vi "Initialize.vi"(8 "error in (no error)":errorcluster, 10 "Name":string, 11 "Filter Wheel Simulator in":refnum<class "Filter Wheel Simulator.lvclass">) -> (0 "error out":errorcluster, 3 "Filter Wheel Simulator out":refnum<class "Filter Wheel Simulator.lvclass">)   [LabVIEW 2021, in "Filter Wheel Simulator.lvclass"]
uses:
  Filter Wheel Simulator.lvclass
  Filter Wheel cluster Simulated Status.ctl
  Filter Wheel Simulator.lvclass/Filter Wheel Simulator.ctl
  Filter Wheel Object/Filter Wheel.lvclass
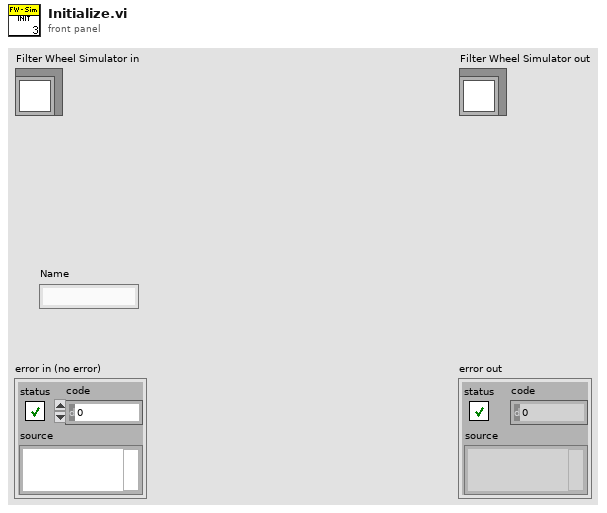
[diagram p1: front panel]
types:
  T1 = typedef "Filter Wheel Simulator.lvclass/Filter Wheel cluster Simulated Status.ctl" = cluster{"Move Start Time":timestamp, "Moving?":bool, "Target Pos":dbl, "Direction":bool}
  T2 = typedef "Filter Wheel.lvclass/Filter Wheel configuration.ctl" = cluster{"Num Wheels":i32, "Filters":T3[], "Invalid Combinations":i32[][], "Addr":refnum<visa-resource-name>, "Name":string, "Simulate":bool, "Homing Parameters":T4, "Default Speed":u16}
  T3 = typedef "Filter Wheel.lvclass/Filter Wheel Details.ctl" = cluster{"Names":string[], "Relative Position":i32[], "Wheel Name":string}
  T4 = typedef "Filter Wheel Arduino Homing cluster.ctl" = cluster{"Direction (F: CW)":bool, "Speed":i32, "Accel":i32, "Min Distance":i32, "Short Leg":i32, "Error Cnts":i32}
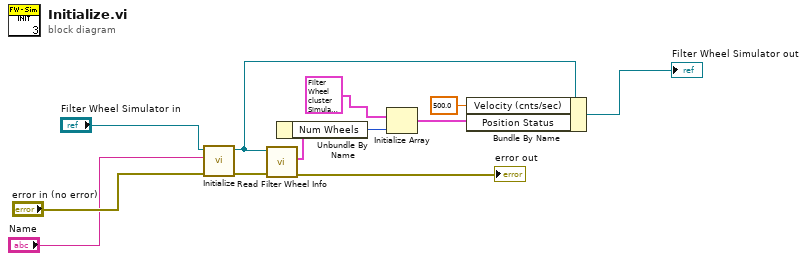
[diagram p0: block diagram]
diagram:
  n1 = call-parent "Initialize.vi"("error in (no error)"="error in (no error)", "Name"="Name", "Filter Wheel in"="Filter Wheel Simulator in") -> ("error out"=w7:errorcluster, "Filter Wheel out"=w8:refnum<class "Filter Wheel Simulator.lvclass">)  [unwired: 7 in]
  n2 = call-dynamic "Read Filter Wheel Info.vi"("error in (no error)"=w7, "Filter Wheel in"=w8) -> ("error out"=→"error out":errorcluster, "Filter Wheel Info"=w6:T2)  [unwired: 7 in, 1 out]
  n3 = Unbundle By Name(w6) -> ("Num Wheels"=w5:i32)
  n4 = Initialize Array(T1 {"Move Start Time"=timestamp(0 s since 1904-01-01), "Moving?"=FALSE, "Target Pos"=0.0, "Direction"=FALSE} ("Position Status"), w5) -> (w3:T1[])
  n5 = Bundle By Name(cluster=w8, "Velocity (cnts/sec)"=500.0, "Position Status"=w3) -> (→"Filter Wheel Simulator out":refnum<class "Filter Wheel Simulator.lvclass">)
